vi "testSendTelToClient.vi"(8 "error in (no error)":errorcluster) -> (0 "error out":errorcluster)   [LabVIEW 2018]
doc: "This VI sends telemetry from TCP client to TCP server."
uses:
  <vilib>/addons/_JKI Toolkits/Caraya/classes/Assert/Assert Equal Value_Variant.vi
  src/TcpServer/TcpServer.lvclass
  <vilib>/addons/_JKI Toolkits/Caraya/classes/Test/Test.lvclass
  <vilib>/addons/_JKI Toolkits/Caraya/classes/Assert/Assert.lvclass
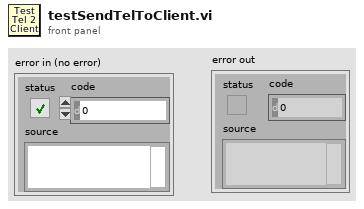
[diagram p1: front panel]
types:
  T1 = typedef "TcpServer.lvclass/userEventTypeDef.ctl" = cluster{"CmdRead":refnum<user-event>, "EvtRead":refnum<user-event>, "GenRead":refnum<user-event>, "ConnStatus":refnum<user-event>}
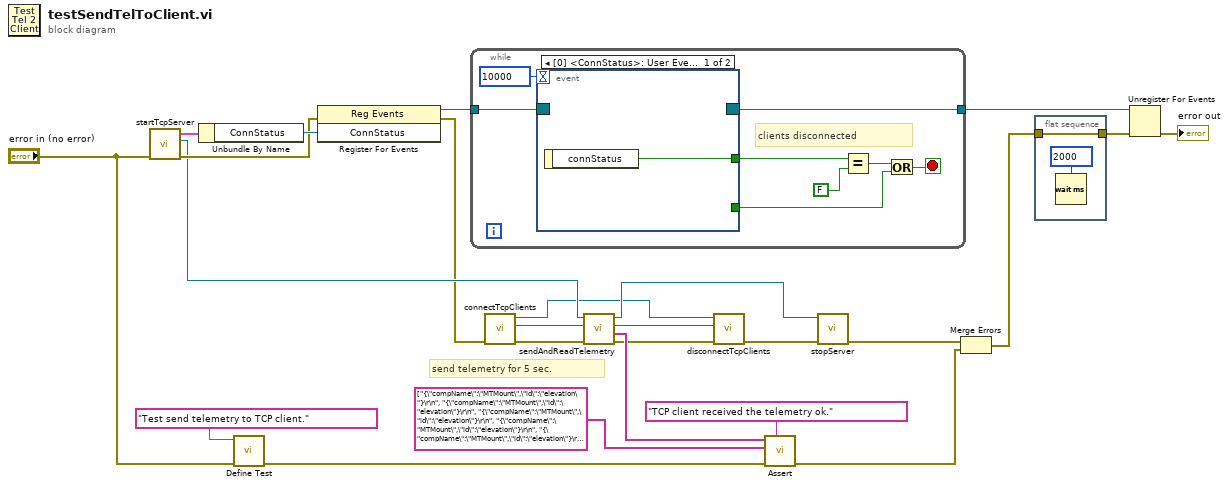
[diagram p0: block diagram]
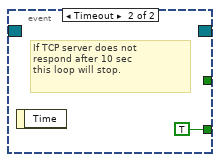
[diagram p2: hidden frame]
diagram:
  # "send telemetry for 5 sec."
  n1 = call "startTcpServer.vi"("error in (no error)"="error in (no error)") -> ("error out"=w19:errorcluster, "TcpServer out"=w9:refnum<class "TcpServer.lvclass">, "User Events"=w21:T1)  [unwired: 8 in]
  n2 = Unbundle By Name(w21) -> ("ConnStatus"=w20:refnum<user-event>)
  n3 = call <vilib>:"Define Test.vi"("error in (no error)"="error in (no error)", "Label (VI Title)"="Test send telemetry to TCP client.") -> ("error out"=w14:errorcluster)  [unwired: 9 in]
  n4 = register-events(error in=w19, w20) -> (reference out=w25:refnum<event-registration>, error out=w1:errorcluster)  [unwired: 1 in]
  n5 = while {
    tunnel: w25 -> [w33]
    tunnel: [w32] -> w24
    stop <- w28 stop-if-true
    # "clients disconnected"
    n6 = event shown="[0] <ConnStatus>: User Event" {
      selector: w33 -> [_ _]
      dyn-events: [_ _] -> w32
      timeout: 10000 -> [_ _]
      tunnel: [w34 _] -> w31
      tunnel: [_ TRUE] -> w27
      event User Event {
        n7 = event-data() -> ("connStatus"=w34:bool)  [unwired: 1 in]
      }
      event Timeout {
        # "If TCP server does not\nrespond after 10 sec\nthis loop will stop."
        n8 = event-data() -> ()  [unwired: 1 in, 1 out]
      }
    }
    n9 = Equal?(x=w31, y=FALSE) -> (x = y?=w29:bool)
    n10 = Or(x=w29, y=w27) -> (x .or. y?=w28:bool)
  }
  n11 = call "connectTcpClients.vi"("error in (no error)"=w1) -> ("error out"=w3:errorcluster, "tel connection ID out"=w5:refnum<k5>, "cmd connection ID out"=w6:refnum<k5>)  [unwired: 8 in]
  n12 = call "sendAndReadTelemetry.vi"("error in (no error)"=w3, "tel connection in"=w5, "TcpServer out"=w9) -> ("error out"=w2:errorcluster, "telemetry received"=w7:string[], "tel connection out"=w4:refnum<k5>, "tcpServer out"=w8:refnum<class "TcpServer.lvclass">)  [unwired: 5 in]
  n13 = call "disconnectTcpClients.vi"("error in (no error)"=w2, "tel connection ID in"=w4, "cmd connection ID in"=w6) -> ("error out"=w18:errorcluster)  [unwired: 8 in]
  n14 = call-poly <vilib>:"Assert.vi"("Label"="TCP client received the telemetry ok.", "error in (no error)"=w14, "Y"=string[] ["{\"compName\":\"MTMount\",\"id\":\"elevation\"}\r\n", "{\"compName\":\"MTMount\",\"id\":\"elevation\"}\r\n", "{\"compName\":\"MTMount\",\"id\":\"elevation\"}\r\n", "{\"compName\":\"MTMount\",\"id\":\"elevation\"}\r\n", "{\"compName\":\"MTMount\",\"id\":\"elevation\"}\r\n", "{\"compName\":\"MTMount\",\"id\":\"elevation\"}\r\n", "{\"compName\":\"MTMount\",\"id\":\"elevation\"}\r\n", "{\"compName\":\"MTMount\",\"id\":\"elevation\"}\r\n", "{\"compName\":\"MTMount\",\"id\":\"elevation\"}\r\n", "{\"compName\":\"MTMount\",\"id\":\"elevation\"}\r\n", "{\"compName\":\"MTMount\",\"id\":\"elevation\"}\r\n", "{\"compName\":\"MTMount\",\"id\":\"elevation\"}\r\n", "{\"compName\":\"MTMount\",\"id\":\"elevation\"}\r\n", "{\"compName\":\"MTMount\",\"id\":\"elevation\"}\r\n", "{\"compName\":\"MTMount\",\"id\":\"elevation\"}\r\n", "{\"compName\":\"MTMount\",\"id\":\"elevation\"}\r\n", "{\"compName\":\"MTMount\",\"id\":\"elevation\"}\r\n", "{\"compName\":\"MTMount\",\"id\":\"elevation\"}\r\n", "{\"compName\":\"MTMount\",\"id\":\"elevation\"}\r\n", "{\"compName\":\"MTMount\",\"id\":\"elevation\"}\r\n", "{\"compName\":\"MTMount\",\"id\":\"elevation\"}\r\n", "{\"compName\":\"MTMount\",\"id\":\"elevation\"}\r\n", "{\"compName\":\"MTMount\",\"id\":\"elevation\"}\r\n", "{\"compName\":\"MTMount\",\"id\":\"elevation\"}\r\n", "{\"compName\":\"MTMount\",\"id\":\"elevation\"}\r\n", "{\"compName\":\"MTMount\",\"id\":\"elevation\"}\r\n", "{\"compName\":\"MTMount\",\"id\":\"elevation\"}\r\n", "{\"compName\":\"MTMount\",\"id\":\"elevation\"}\r\n", "{\"compName\":\"MTMount\",\"id\":\"elevation\"}\r\n", "{\"compName\":\"MTMount\",\"id\":\"elevation\"}\r\n", "{\"compName\":\"MTMount\",\"id\":\"elevation\"}\r\n", "{\"compName\":\"MTMount\",\"id\":\"elevation\"}\r\n", "{\"compName\":\"MTMount\",\"id\":\"elevation\"}\r\n", "{\"compName\":\"MTMount\",\"id\":\"elevation\"}\r\n", "{\"compName\":\"MTMount\",\"id\":\"elevation\"}\r\n", "{\"compName\":\"MTMount\",\"id\":\"elevation\"}\r\n", "{\"compName\":\"MTMount\",\"id\":\"elevation\"}\r\n", "{\"compName\":\"MTMount\",\"id\":\"elevation\"}\r\n", "{\"compName\":\"MTMount\",\"id\":\"elevation\"}\r\n", "{\"compName\":\"MTMount\",\"id\":\"elevation\"}\r\n", "{\"compName\":\"MTMount\",\"id\":\"elevation\"}\r\n", "{\"compName\":\"MTMount\",\"id\":\"elevation\"}\r\n", "{\"compName\":\"MTMount\",\"id\":\"elevation\"}\r\n", "{\"compName\":\"MTMount\",\"id\":\"elevation\"}\r\n", "{\"compName\":\"MTMount\",\"id\":\"elevation\"}\r\n", "{\"compName\":\"MTMount\",\"id\":\"elevation\"}\r\n", "{\"compName\":\"MTMount\",\"id\":\"elevation\"}\r\n", "{\"compName\":\"MTMount\",\"id\":\"elevation\"}\r\n", "{\"compName\":\"MTMount\",\"id\":\"elevation\"}\r\n", "{\"compName\":\"MTMount\",\"id\":\"elevation\"}\r\n"] ("Array 2"), "X"=w7) -> ("error out"=w11:errorcluster)  [unwired: 7 in]
  n15 = call "stopServer.vi"("error in (no error)"=w18, "tcpServer in"=w8) -> ("error out"=w12:errorcluster)  [unwired: 8 in, 1 out]
  n16 = Merge Errors(w12, w11) -> (w10:errorcluster)
  n17 = flat-sequence {
    tunnel: w10 -> [w36]
    tunnel: [w36] -> w22
    frame #0 {
      n18 = Wait (ms)(milliseconds to wait=u32 2000) -> ()  [unwired: 1 out]
    }
  }
  n19 = Unregister For Events(event registration refnum=w24, error in=w22) -> (error out=→"error out":errorcluster)
